vi "read_attributes.vi"(8 "error in (no error)":errorcluster, 11 "ComplementNB in":refnum<class "ComplementNB.lvclass">) -> (0 "error out":errorcluster, 2 "attributes":T1, 3 "ComplementNB out":refnum<class "ComplementNB.lvclass">)   [LabVIEW 2020, in "ComplementNB.lvclass"]
uses:
  ComplementNB.lvclass
  Controls/complement_nb_attributes.ctl
  ComplementNB.lvclass/ComplementNB.ctl
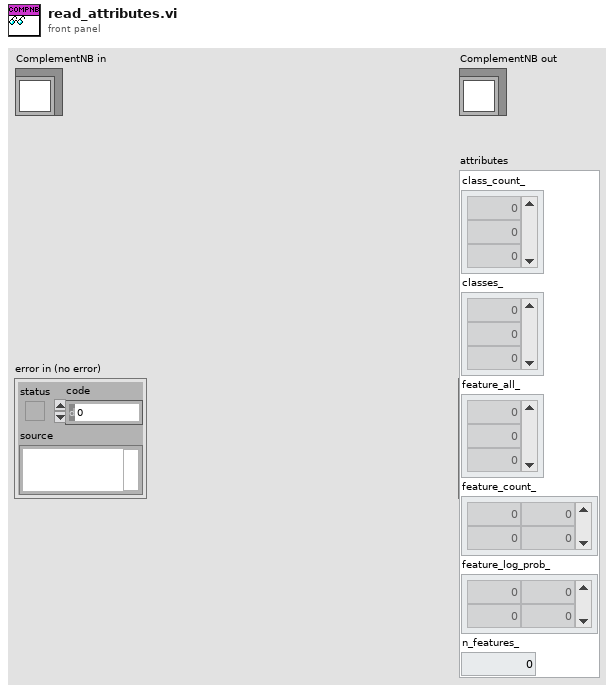
[diagram p1: front panel]
types:
  T1 = typedef "complement_nb_attributes.ctl" = cluster{"class_count_":dbl[], "classes_":dbl[], "feature_all_":dbl[], "feature_count_":dbl[][], "feature_log_prob_":dbl[][], "n_features_":dbl}
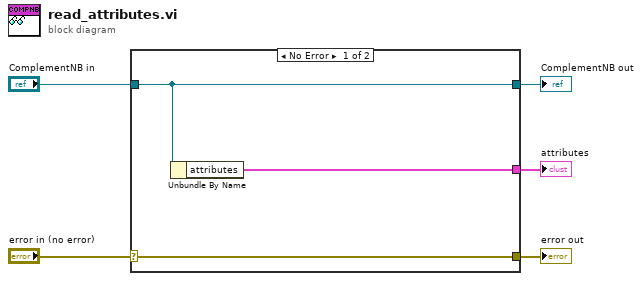
[diagram p0: block diagram]
diagram:
  n1 = case shown="No Error" "error in (no error)" {
    selector: "error in (no error)" -> [w8 w9]
    tunnel: [w8 w9] -> w4
    tunnel: [w7 w10] -> w2
    tunnel: "ComplementNB in" -> [w7 w10]
    tunnel: [w6 _] -> w1
    frame No Error {
      n2 = Unbundle By Name(w7) -> ("attributes"=w6:T1)
    }
    frame Error {
    }
  }
  "error out" <- w4
  "ComplementNB out" <- w2
  "attributes" <- w1
